vi "Make File Read-Only.vi"(8 "error in (no error)":errorcluster, 11 "File Path in":path) -> (0 "error out":errorcluster, 3 "File Path out":path)   [LabVIEW 2015, in "Segmented Log.lvclass"]
uses:
  Segmented Log.lvclass
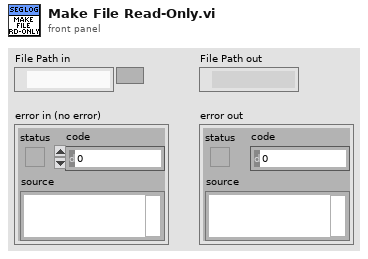
[diagram p1: front panel]
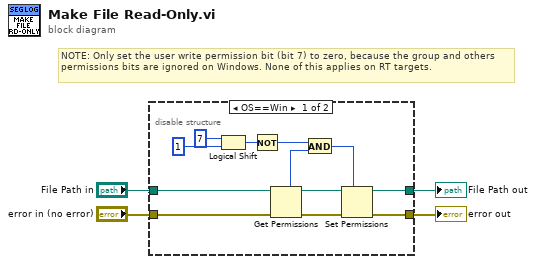
[diagram p0: block diagram]
diagram:
  # "NOTE: Only set the user write permission bit (bit 7) to zero, because the group and others permissions bits are ignored on Windows. None of this applies on RT targets."
  n1 = disable-structure shown="OS==Win" {
    disable-tunnel: [w16 w18] -> w4
    disable-tunnel: [w15 w17] -> w3
    disable-tunnel: "error in (no error)" -> [w13 w17]
    disable-tunnel: "File Path in" -> [w12 w18]
    frame condition #0 (active) {
      n2 = Logical Shift(y=i8 7, x=i16 1) -> (x << y=w6:i16)
      n3 = Not(x=w6) -> (.not. x?=w5:i16)
      n4 = Get Permissions(8:w13, 11:w12) -> (0:w14:errorcluster, 3:w11:path, 5:w10:i16)  [unwired: 2 out]
      n5 = And(x=w5, y=w10) -> (x .and. y?=w9:i16)
      n6 = Set Permissions(7:w9, 8:w14, 11:w11) -> (0:w15:errorcluster, 3:w16:path)  [unwired: 2 in]
    }
    frame condition #1 {
      # "Setting file permissions not applicable on PharLap/VxWorks."
    }
  }
  "File Path out" <- w4
  "error out" <- w3
